vi "EXTRACT-DATA-UINT8.vi"(2 "UINT8":u8, 7 "Data":u8[](array[numeric])) -> (4 "Value":u8, 8 "Min":u8, 10 "Max":u8, 15 "Inc":u8)   [LabVIEW 2019]
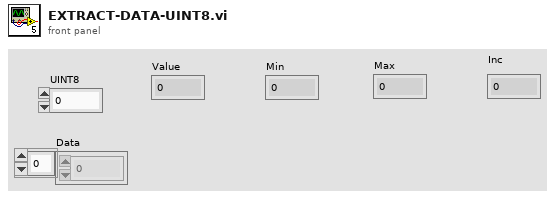
[diagram p1: front panel]
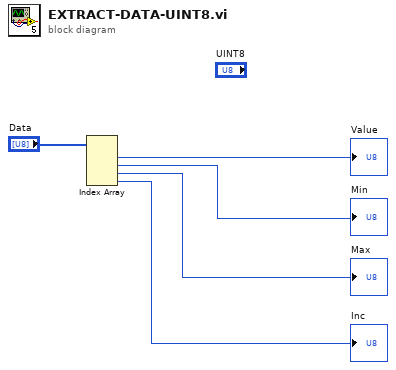
[diagram p0: block diagram]
diagram:
  n1 = Index Array(array="Data") -> (element #1=→"Value":u8, element #2=→"Min":u8, element #3=→"Max":u8, element #4=→"Inc":u8)  [unwired: 4 in]
